vi "Write INIndex.vi"(8 "error in (no error)":errorcluster, 10 "INIndex":i32, 11 "AI in":refnum<class "AI.lvclass">) -> (0 "error out":errorcluster, 3 "AI out":refnum<class "AI.lvclass">)   [LabVIEW 2019, in "AI.lvclass"]
uses:
  AI.lvclass
  FlowIOCtrl.lvclass
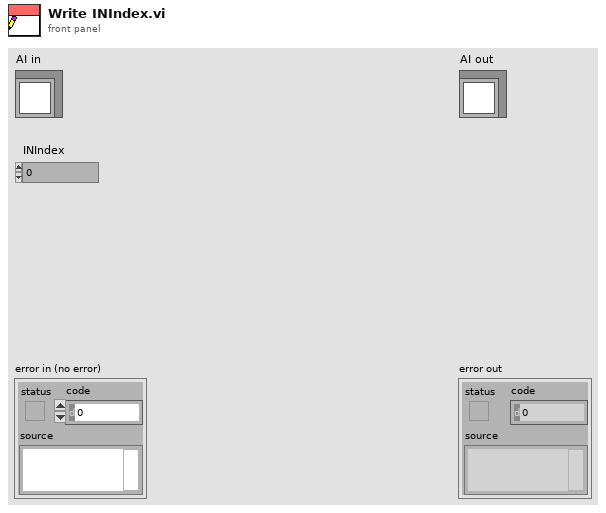
[diagram p1: front panel]
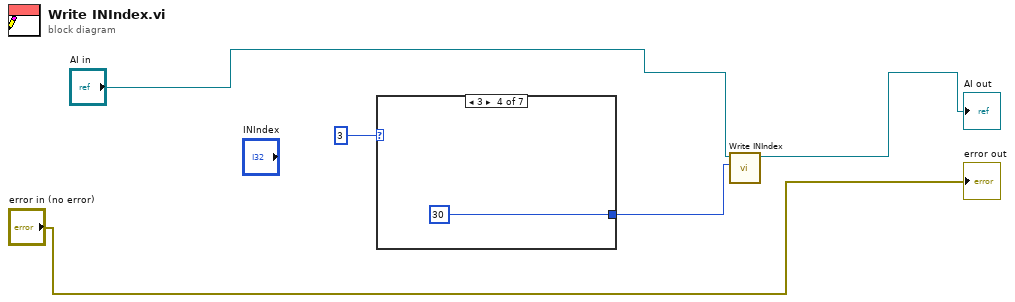
[diagram p0: block diagram]
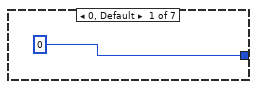
[diagram p2: hidden frame]
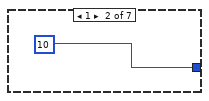
[diagram p3: hidden frame]
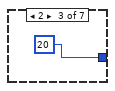
[diagram p4: hidden frame]
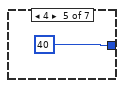
[diagram p5: hidden frame]
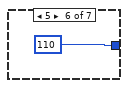
[diagram p6: hidden frame]
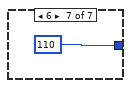
[diagram p7: hidden frame]
diagram:
  n1 = case shown="3" 3 {
    tunnel: [0 10 20 30 40 110 110 ("ModbusIOInput")] -> w2
    frame 0, Default {
    }
    frame 1 {
    }
    frame 2 {
    }
    frame 3 {
    }
    frame 4 {
    }
    frame 5 {
    }
    frame 6 {
    }
  }
  n2 = call-parent "Write INIndex.vi"("INIndex"=w2, "Station Action in"="AI in") -> ("Station Action out"=→"AI out":refnum<class "AI.lvclass">)  [unwired: 8 in, 1 out]
  "error out" <- "error in (no error)"
